vi "SaveWaveformToFile.vi"(8 "error in (no error)":errorcluster, 10 "Waveform":waveform(dbl), 11 "Byte Stream File in":refnum<file>) -> (0 "error out":errorcluster, 3 "Byte Stream File out":refnum<file>)   [LabVIEW 2022 SP3]
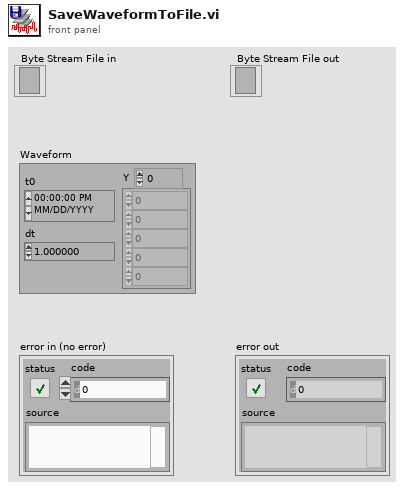
[diagram p1: front panel]
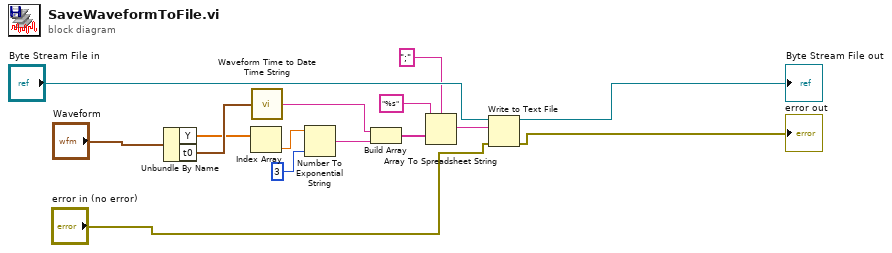
[diagram p0: block diagram]
diagram:
  n1 = Unbundle By Name("Waveform") -> ("Y"=w2:dbl[], "t0"=w7:timestamp)
  n2 = Index Array(array=w2) -> (element=w4:dbl)  [unwired: 1 in]
  n3 = call <vilib>:"Waveform Time to Date Time String.vi"("t0"=w7) -> ("String"=w6:string)
  n4 = Number To Exponential String(number=w4, precision (6)=i16 3) -> (E-format string=w3:string)  [unwired: 2 in]
  n5 = Build Array(w6, w3) -> (w9:string[])
  n6 = Array To Spreadsheet String(delimiter (Tab)=";", array=w9, 3:"%s" ("format string")) -> (spreadsheet string=w10:string)
  n7 = Write to Text File(file (use dialog)="Byte Stream File in", text=w10, error in="error in (no error)") -> (refnum out=→"Byte Stream File out":refnum<file>, error out=→"error out":errorcluster)  [unwired: 1 in, 1 out]
